vi "Encode Array.vi"(7 "Delimiter (\",\")":string=",", 11 "1D Array in":string[](array[string])) -> (3 "JSON out":string)   [LabVIEW 2019, in "JSON.lvlib"]
uses:
  JSON.lvlib
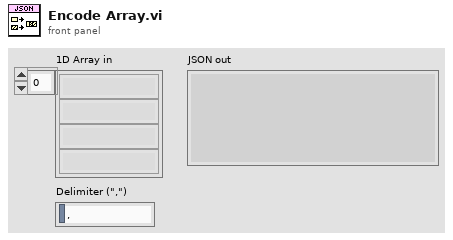
[diagram p1: front panel]
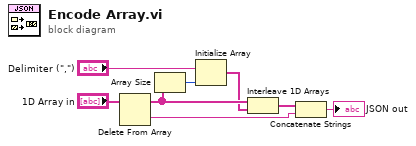
[diagram p0: block diagram]
diagram:
  n1 = Delete From Array(array="1D Array in") -> (deleted portion=w1:string, array with subset deleted=w3:string[])  [unwired: 2 in]
  n2 = Array Size(array=w3) -> (size(s)=w5:i32)
  n3 = Initialize Array("Delimiter (\",\")", w5) -> (w2:string[])
  n4 = Interleave 1D Arrays(w3, w2) -> (w8:string[])
  n5 = Concatenate Strings(w8, w1) -> (→"JSON out":string)
